vi "Sgl_to_Half_Prec_Poly.vi"   [LabVIEW 2015]
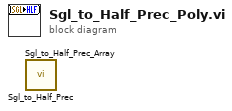
[diagram p0: block diagram]
diagram:
  n1 = call "Sgl_to_Half_Prec.vi"() -> ()  [unwired: 5 in, 1 out]
  n2 = call "Sgl_to_Half_Prec_Array.vi"() -> ()  [unwired: 5 in, 1 out]
